vi "Definition Cluster.vi"(11 "Entity in":refnum<class "Entity.lvclass">) -> (2 "Definition":variant, 3 "Entity out":refnum<class "Entity.lvclass">)   [LabVIEW 2020, in "Conditu2.lvlib" / "Columns.lvlib" / "Entity.lvclass"]
uses:
  Entity.lvclass
  C:/dev/lv20CE/lv-conditum-tools/Conditum-Clone/Columns/Relation/Relation.lvclass
  Relation/Relation Definition.ctl
  Type/Definition.ctl
  Relation/Relation Info.ctl
  Relation Mapping.ctl
  Conditu2.lvlib
  Relation/Relation.lvclass
  Type/Type.lvclass
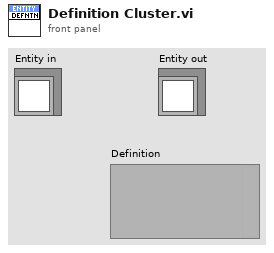
[diagram p1: front panel]
types:
  T1 = typedef "Conditu2.lvlib/Columns.lvlib/Relation.lvclass/Relation Definition.ctl" = cluster{"Type":T2, "Relation":T3}
  T2 = typedef "Conditu2.lvlib/Columns.lvlib/Type.lvclass/Definition.ctl" = cluster{"Name":string, "Nullable":bool, "Default NULL":bool}
  T3 = typedef "Conditu2.lvlib/Relation Info.ctl" = cluster{"Mapping":T4, "Related To":string, "Reversed By":string}
  T4 = typedef "Conditu2.lvlib/Relation Mapping.ctl" = enum16{"OneToOne", "OneToMany", "ManyToOne", "ManyToMany"}
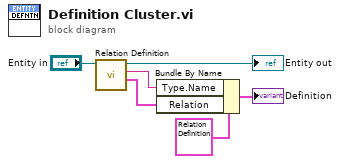
[diagram p0: block diagram]
diagram:
  n1 = call "Relation Definition.vi"("Relation in"="Entity in") -> ("Relation Definition"=w4:T3, "Table Name"=w5:string, "Relation out"=→"Entity out":refnum<class "Entity.lvclass">)  [unwired: 8 in]
  n2 = Bundle By Name(cluster=T1 {"Type"={"Name"="", "Nullable"=FALSE, "Default NULL"=FALSE}, "Relation"={"Mapping"=enum."OneToMany", "Related To"="", "Reversed By"=""}} ("Relation Definition"), "Type.Name"=w5, "Relation"=w4) -> (→"Definition":T1)
